vi "Initialize Controls to default.vi"(8 "error in (no error)":errorcluster, 11 "VI in":refnum<vi>) -> (0 "error out":errorcluster)   [LabVIEW 2016]
doc: "Change current values of all controls on the front panel to their defaults."
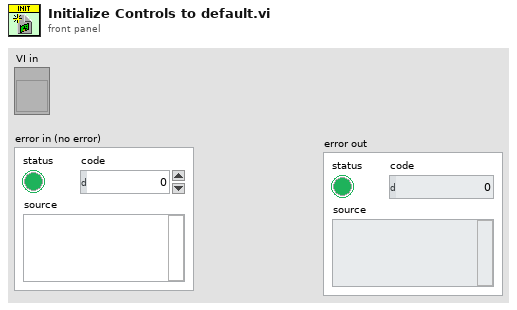
[diagram p1: front panel]
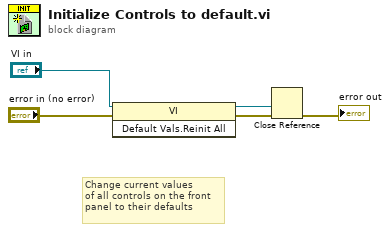
[diagram p0: block diagram]
diagram:
  # "Change current values\nof all controls on the front\npanel to their defaults"
  n1 = invoke class="VI" method="Default Vals.Reinit All"(reference="VI in", error in="error in (no error)") -> (reference out=w3:refnum<vi>, error out=w4:errorcluster)  [unwired: 1 in, 1 out]
  n2 = Close Reference(reference=w3, error in (no error)=w4) -> (error out=→"error out":errorcluster)
